vi "Check_Execution_Row.vi"(0 "Execution Row":T1 {"Row Duration (mins)" format="%#.1f"; "Row No" min=0; "Trace Gas Concentration (%)" min=0.0 format="%#.2f"; "Emission Rate (l/min)" format="%#.2f"; "Tunnel Speed" format="%#.2f"; "Start X" format="%#.2f"; "Start Y" format="%#.2f"; "Start Z" format="%#.2f"; "End X" format="%#.2f"; "End Y" format="%#.2f"; "End Z" format="%#.2f"; "Averaging time (min)" min=0.0 format="%#.2f"}, 3 "Synchronization Start No":i32=1 min=1 max=100, 4 "Row Index":i32, 5 "Max Tunnel Speed":dbl format="%.2f") -> (6 "Editted Row":bool, 7 "Execution Row Out":T1 {"Row Duration (mins)" format="%#.1f"; "Row No" min=0; "Trace Gas Concentration (%)" min=0.0 format="%#.2f"; "Emission Rate (l/min)" format="%#.2f"; "Tunnel Speed" format="%#.2f"; "Start X" format="%#.2f"; "Start Y" format="%#.2f"; "Start Z" format="%#.2f"; "End X" format="%#.2f"; "End Y" format="%#.2f"; "End Z" format="%#.2f"; "Averaging time (min)" min=0.0 format="%#.2f"}, 9 "Continue?":bool, 10 "Error Comments":string)   [LabVIEW 2011]
uses:
  Traverse_cluster.ctl
  Spacing.ctl
  Controls/Multi_run_mode.ctl
  Controls/User_Specific_mode.ctl
  Controls/Tunnel_Coordinates.ctl
  ADAM Client/Sub VIs/ADAM Controls/Channel_names.ctl
  Globals/Extra_Commands_Global.vi
  Globals/Constants_global.vi
  Globals/Trav_pos_global.vi
panel:
  out "Fixed Axis":bool[](array[boolean])
  out "Filenames":string[](array[string])
  out "Current Sync Number":i32
  out "Checks":string[](array[string])
  in  "Edit in Excel":bool
  in  "OK":bool
  # "X           Y            Z"
  # "Start"
  # "End"
  # "X           Y            Z"
  # "Start"
  # "End"
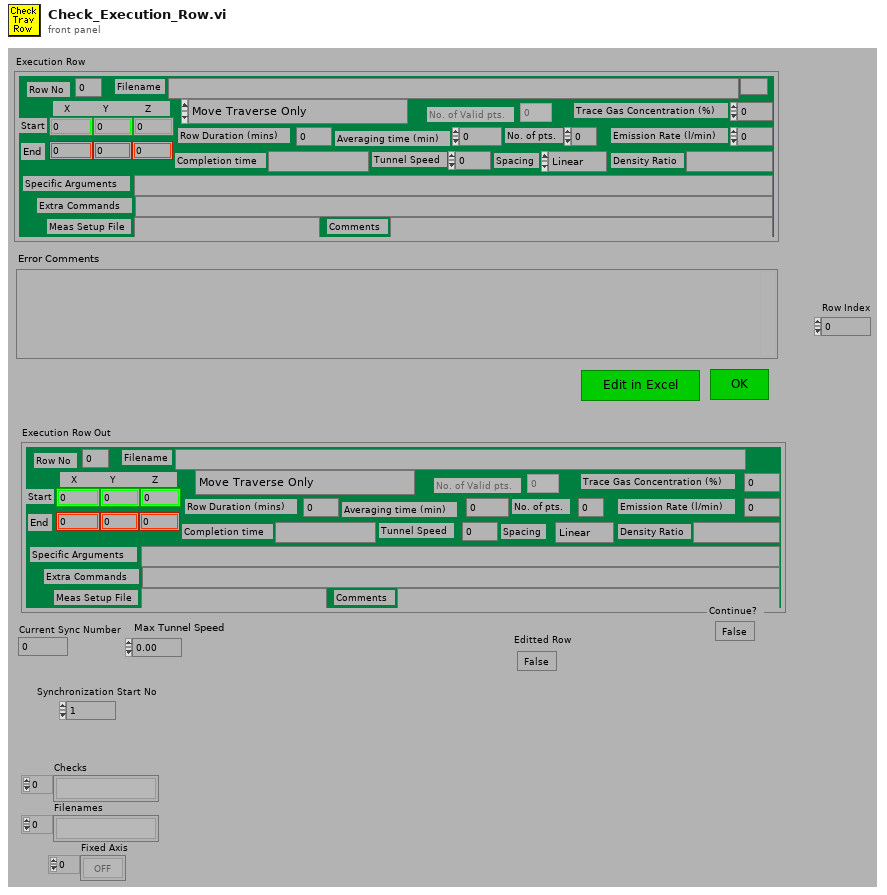
[diagram p1: front panel]
types:
  T1 = typedef "Traverse_cluster.ctl" = cluster{"Start X":dbl, "Start Y":dbl, "Start Z":dbl, "End X":dbl, "End Y":dbl, "End Z":dbl, "No. of pts.":i32, "Spacing":T2, "Filename":path, "Tunnel Speed":dbl, "Averaging time (min)":dbl, "Extra Commands":string, "Specific Arguments":string, "Emission Rate (l/min)":dbl, "Trace Gas Concentration (%)":dbl, "Density Ratio":string, "Comments":string, "Row No":i32, "Row Type Selector":T3, "Completion time":string, "Row Duration (mins)":dbl, "No. of Valid pts.":i32, "Meas Setup File":string}
  T2 = typedef "Spacing.ctl" = enum16{"Linear", "Log", "Gauss", "Specified", "N/A"}
  T3 = typedef "Multi_run_mode.ctl" = enum16{"Move Traverse Only", "Set Tunnel Speed Only", "Set Source Only", "Set Measurement Conditions", "Single Measurement", "Vertical Profile", "Lateral Profile", "Longitudinal Profile", "Explore Volume", "Multi-Axis Profile", "Auto Calibrate", "Meas Fast FID Bkgnd", "Check Beam Power", "Scanning Valve Measurement", "Run VI Named:", "Set ADAM Ch", "Wait (minutes)", "Send Message", "Synchronize With:", "Fall Back to this Row", "Turn Off Row Repeating", "Blank Row"}
  T4 = enum16{"All Channel Names", "Valid Channel Names"}
  T5 = typedef "User_Specific_mode.ctl" = enum16{"Check VI only", "Run VI"}
  T6 = typedef "Tunnel_Coordinates.ctl" = enum16{"Work in Tunnel Coordinates", "Work in Model Coordinates"}
  T7 = enum16{"Zero or one", "One", "Zero or more", "One or more"}
  T8 = typedef "Channel_names.ctl" = enum16{"Active Only", "Active + Off", "All Channels"}
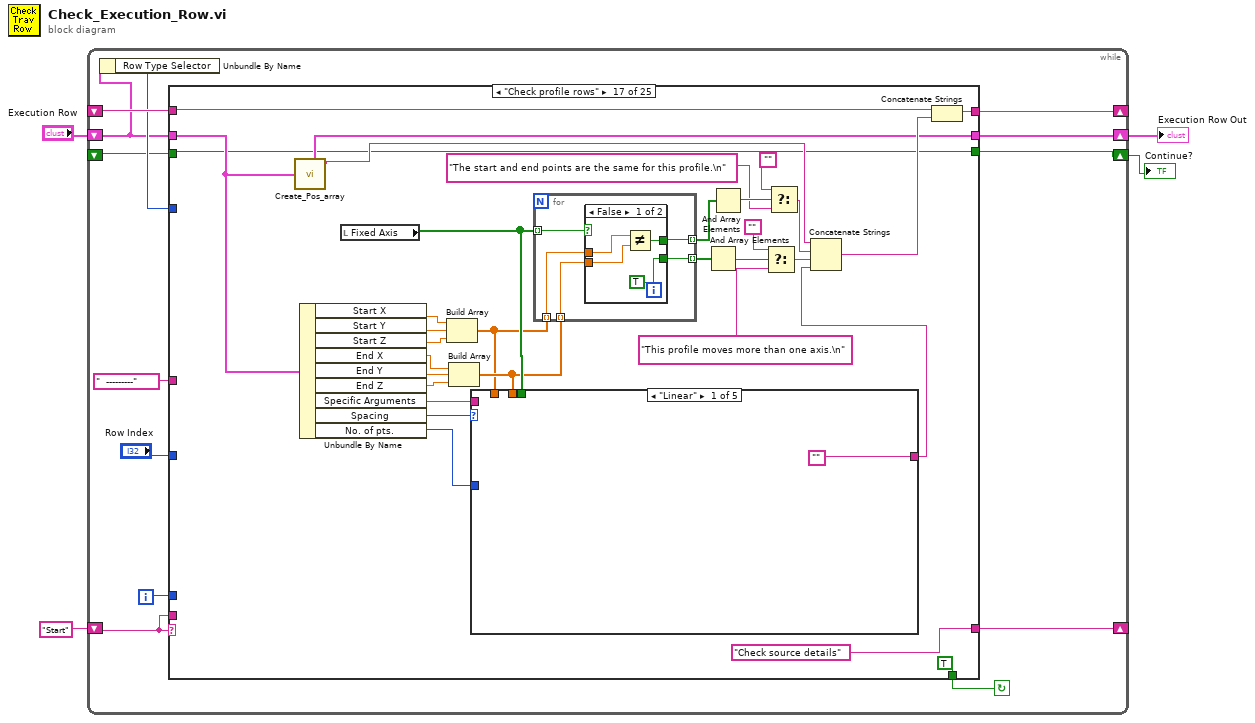
[diagram p0: block diagram]
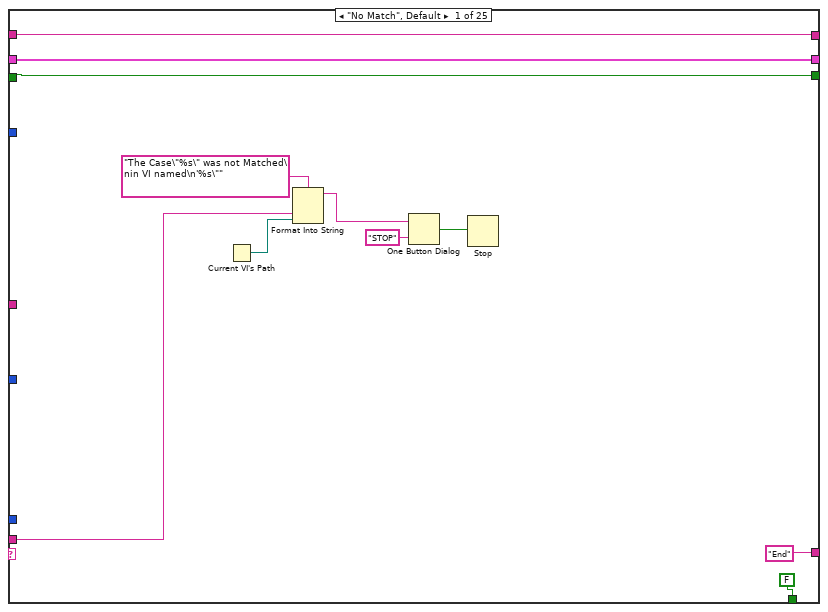
[diagram p2: hidden frame]
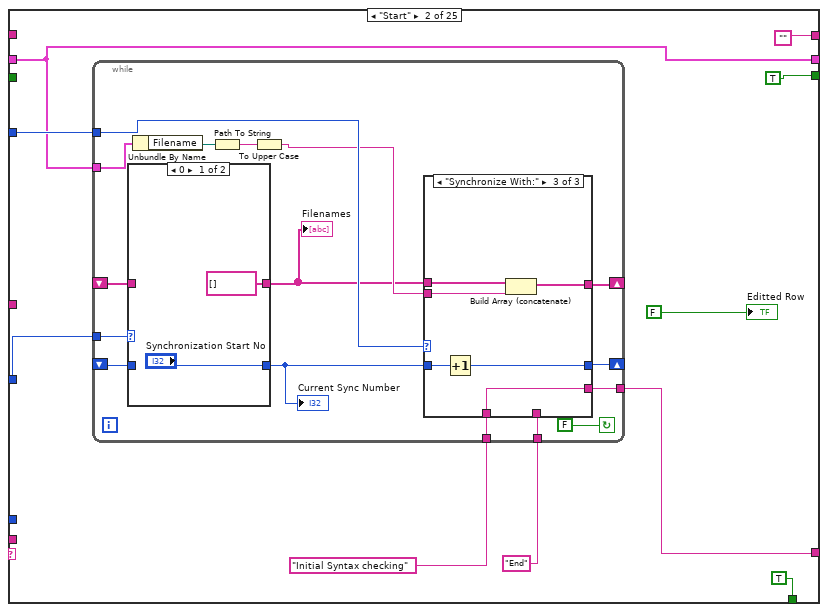
[diagram p3: hidden frame]
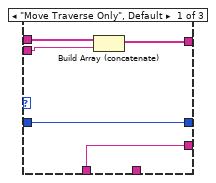
[diagram p5: hidden frame]
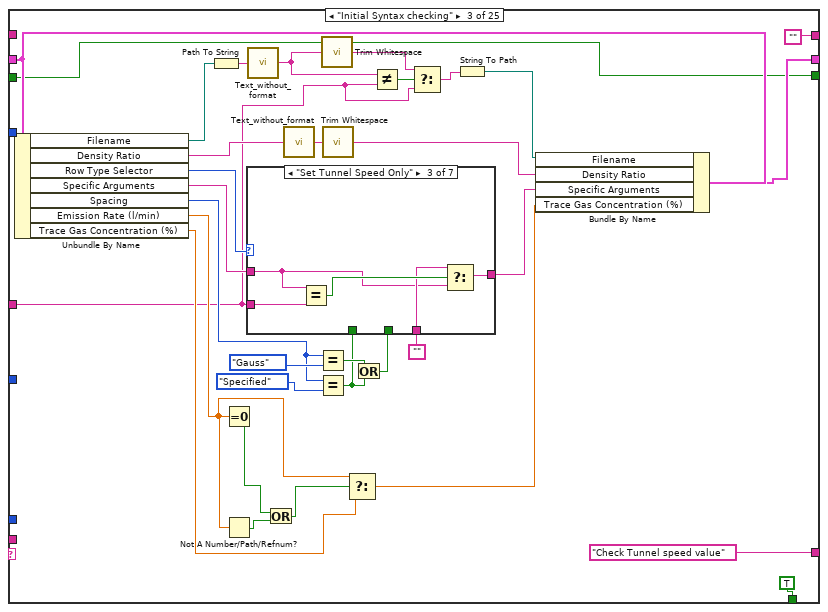
[diagram p7: hidden frame]
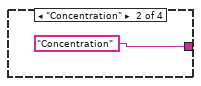
[diagram p10: hidden frame]
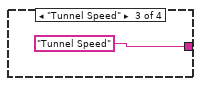
[diagram p11: hidden frame]
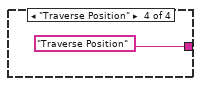
[diagram p12: hidden frame]
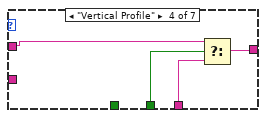
[diagram p13: hidden frame]
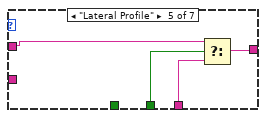
[diagram p14: hidden frame]
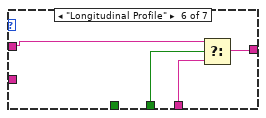
[diagram p15: hidden frame]
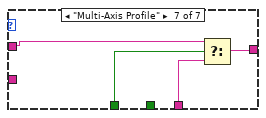
[diagram p16: hidden frame]
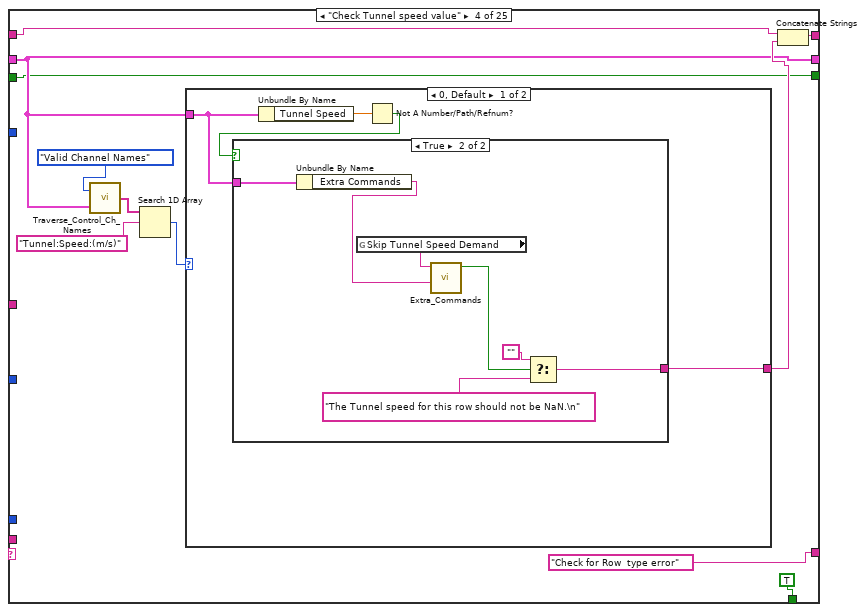
[diagram p17: hidden frame]
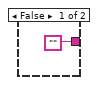
[diagram p18: hidden frame]
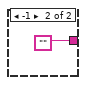
[diagram p19: hidden frame]
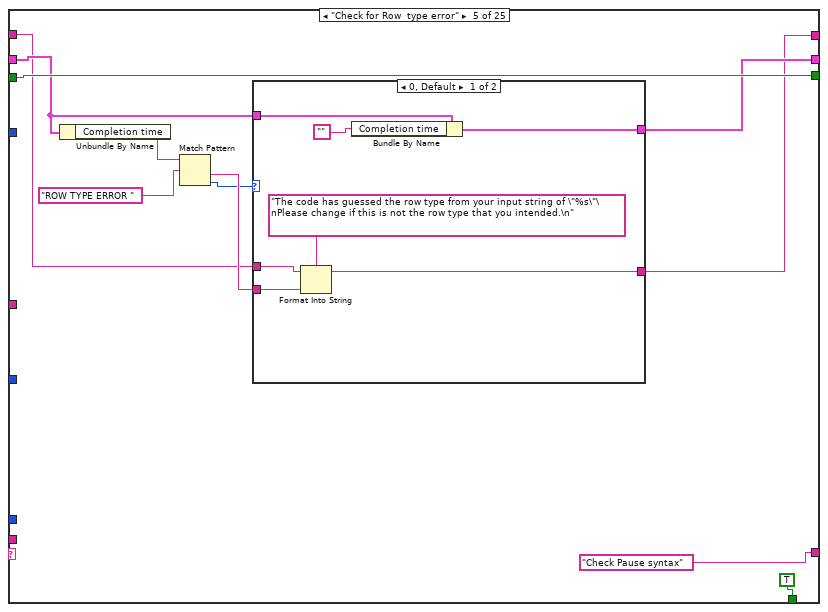
[diagram p20: hidden frame]
diagram:
  n1 = while {
    shift-left: _ -> [w16]
    shift-right: [w17] -> _
    shift-left: "Start" -> [w9]
    shift-right: [w14] -> _
    shift-right: [w8] -> w2
    shift-left: "Execution Row" -> [w5]
    shift-right: [w7] -> w1
    shift-left: _ -> [w6]
    i -> [w10]
    stop <- w15 continue-if-true
    n2 = Unbundle By Name(w5) -> ("Row Type Selector"=w12:T3)
    n3 = case shown="\"Check profile rows\"" w9 {
      tunnel: w5 -> [w22 w32 w100 w137 w161 w191 w205 w248 w278 w334 w366 w374 w413 w744 w844 w881 w903 w987 w1019 w1029 w1098 _ w1137 w1144 w1154]
      tunnel: "  ---------" ("f") -> [_ _ w74 _ _ w195 _ _ _ _ _ _ _ _ _ _ _ _ _ _ _ _ _ _ _]
      tunnel: "Row Index" -> [_ w36 _ _ _ _ w202 _ _ _ _ _ w407 _ _ _ _ _ _ _ _ _ w1138 _ w1153]
      tunnel: [w21 "" "" w138 w158 w183 w213 w253 w283 w336 w370 w379 w417 w749 w854 w887 w928 w985 w1023 w1030 w1104 w1115 w1139 w1149 w1156] -> w17
      tunnel: w12 -> [_ w35 _ _ _ _ _ _ _ _ _ w377 w416 w745 w842 _ _ _ _ w1034 _ _ _ _ _]
      tunnel: w16 -> [w21 _ _ w139 w159 w185 w214 w254 w284 w336 w369 w380 w418 w749 w855 w888 w929 w985 w1024 w1035 w1104 w1115 w1139 w1149 w1156]
      tunnel: [FALSE TRUE TRUE TRUE TRUE TRUE TRUE TRUE TRUE TRUE TRUE TRUE TRUE TRUE TRUE TRUE TRUE TRUE TRUE w1026 TRUE TRUE TRUE TRUE FALSE] -> w15
      tunnel: ["End" w33 "Check Tunnel speed value" ("f") "Check for Row  type error" ("f") "Check Pause syntax" ("f") w188 "Check Traverse Setup Name" ("f") "Check IF command" ("f") "Check Measurement Setup?" ("f") w338 "Check Maximum tunnel speed" ("f") "Row type specific check" ("f") w414 "Check for position NaNs" ("f") w845 "Check source details" ("t") "Check source details" ("f") w982 "check entered filename etc" ("f") w1032 "What to do next?" ("f") w1113 "Initial Syntax checking" "End" "End"] -> w14
      tunnel: w10 -> [_ _ _ _ _ _ _ _ _ _ _ _ _ _ _ _ _ _ _ _ _ _ _ _ _]
      tunnel: w9 -> [w23 _ _ _ _ _ _ _ _ _ _ _ _ _ _ _ _ _ _ _ _ _ _ _ _]
      tunnel: [w22 w32 w77 w137 w162 w178 w204 w248 w278 w334 w365 w374 w408 w743 w844 w881 w902 w986 w1019 w1028 w1098 w1106 w1140 w1144 w1152] -> w8
      tunnel: [w18 TRUE w75 w136 w168 w179 w206 w245 w275 w340 w367 w372 w410 w741 w843 w880 w900 w990 w1017 w1026 w1097 w1105 w1134 w1143 w1150] -> w7
      tunnel: w6 -> [w18 _ w75 w136 w168 w179 w206 w245 w275 w340 w367 w372 w410 w741 w843 w880 w900 w990 w1017 _ w1097 _ w1134 w1143 w1150]
      frame "No Match", Default {
        n4 = Current VI's Path() -> (path=w24:path)
        n5 = Format Into String(format string="The Case\"%s\" was not Matched\nin VI named\n'%s\"" ("Format String"), w23, w24) -> (resulting string=w27:string)  [unwired: 2 in, 1 out]
        n6 = One Button Dialog(message=w27, button name ("OK")="STOP") -> (true=w25:bool)
        n7 = Stop(stop? (T)=w25) -> ()
      }
      frame "Start" {
        n8 = while {
          tunnel: "End" -> [w40]
          tunnel: "Initial Syntax checking" -> [w41]
          tunnel: [w42] -> w33
          tunnel: w32 -> [w49]
          shift-left: _ -> [w48]
          shift-right: [w47] -> _
          tunnel: w35 -> [w53]
          shift-left: _ -> [w52]
          shift-right: [w51] -> _
          tunnel: w36 -> [w54]
          stop <- FALSE continue-if-true
          n9 = case shown="0" w54 {
            tunnel: ["Synchronization Start No" w58] -> w50
            tunnel: w52 -> [_ w58]
            tunnel: w48 -> [_ w57]
            tunnel: [string[] [] w57] -> w43
            frame 0 {
            }
            frame 1, Default {
            }
          }
          "Current Sync Number" <- w50
          "Filenames" <- w43
          n10 = Unbundle By Name(w49) -> ("Filename"=w46:path)
          n11 = Path To String(path=w46) -> (string=w45:string)
          n12 = To Upper Case(1:w45) -> (0:w44:string)
          n13 = case shown="\"Synchronize With:\"" w53 {
            tunnel: w50 -> [w63 w66 w72]
            tunnel: [w63 w66 w71] -> w51
            tunnel: w44 -> [w61 _ w70]
            tunnel: w43 -> [w62 w65 w69]
            tunnel: [w60 w65 w68] -> w47
            tunnel: [w59 w64 w67] -> w42
            tunnel: w41 -> [w59 _ w67]
            tunnel: w40 -> [_ w64 _]
            frame "Move Traverse Only", Default {
              n14 = Build Array (concatenate)(w62, w61) -> (w60:string[])
            }
            frame "Blank Row" {
            }
            frame "Synchronize With:" {
              n15 = Increment(x=w72) -> (x+1=w71:i32)
              n16 = Build Array (concatenate)(w69, w70) -> (w68:string[])
            }
          }
        }
        "Editted Row" <- FALSE ("Editted Row")
      }
      frame "Initial Syntax checking" {
        n17 = Unbundle By Name(w100) -> ("Filename"=w73:path, "Density Ratio"=w79:string, "Row Type Selector"=w97:T3, "Specific Arguments"=w95:string, "Spacing"=w87:T2, "Emission Rate (l/min)"=w83:dbl, "Trace Gas Concentration (%)"=w93:dbl)
        n18 = Path To String(path=w73) -> (string=w81:string)
        n19 = Equal To 0?(x=w83) -> (x = 0?=w85:bool)
        n20 = Not A Number/Path/Refnum?(number/path/refnum=w83) -> (NaN/Path/Refnum?=w84:bool)
        n21 = call "Text_without_format.vi"("Input string"=w81) -> ("Output string"=w104:string)
        n22 = Or(x=w85, y=w84) -> (x .or. y?=w82:bool)
        n23 = call "Text_without_format.vi"("Input string"=w79) -> ("Output string"=w99:string)
        n24 = Equal?(x=w87, y=Spacing."Gauss" ("Spacing")) -> (x = y?=w89:bool)
        n25 = Equal?(x=w87, y=Spacing."Specified" ("Spacing")) -> (x = y?=w86:bool)
        n26 = call <vilib>:"Trim Whitespace.vi"("string"=w104) -> ("trimmed string"=w103:string)  [unwired: 1 in]
        n27 = call <vilib>:"Trim Whitespace.vi"("string"=w99) -> ("trimmed string"=w78:string)  [unwired: 1 in]
        n28 = Select(t=w83, s=w82, f=w93) -> (s? t:f=w92:dbl)
        n29 = Or(x=w89, y=w86) -> (x .or. y?=w88:bool)
        n30 = case shown="\"Set Tunnel Speed Only\"" w97 {
          tunnel: [w106 w108 w113 w119 w123 w127 w131] -> w96
          tunnel: w95 -> [w106 w107 w114 w121 w125 w129 w133]
          tunnel: "" -> [_ _ w115 w120 w124 w128 w132]
          tunnel: w88 -> [_ _ _ w118 w122 w126 _]
          tunnel: w86 -> [_ _ _ _ _ _ w130]
          tunnel: w74 -> [_ _ w117 _ _ _ _]
          frame "Move Traverse Only", Default {
          }
          frame "Auto Calibrate" {
            n31 = case shown="\"No Match\", Default" w107 {
              tunnel: [w109 "Concentration" "Tunnel Speed" "Traverse Position"] -> w108
              tunnel: w107 -> [w109 _ _ _]
              frame "No Match", Default {
              }
              frame "Concentration" {
              }
              frame "Tunnel Speed" {
              }
              frame "Traverse Position" {
              }
            }
          }
          frame "Set Tunnel Speed Only" {
            n32 = Equal?(x=w114, y=w117) -> (x = y?=w116:bool)
            n33 = Select(t=w115, s=w116, f=w114) -> (s? t:f=w113:string)
          }
          frame "Vertical Profile" {
            n34 = Select(t=w121, s=w118, f=w120) -> (s? t:f=w119:string)
          }
          frame "Lateral Profile" {
            n35 = Select(t=w125, s=w122, f=w124) -> (s? t:f=w123:string)
          }
          frame "Longitudinal Profile" {
            n36 = Select(t=w129, s=w126, f=w128) -> (s? t:f=w127:string)
          }
          frame "Multi-Axis Profile" {
            n37 = Select(t=w133, s=w130, f=w132) -> (s? t:f=w131:string)
          }
        }
        n38 = Not Equal?(x=w104, y=w74) -> (x != y?=w105:bool)
        n39 = Select(t=w103, s=w105, f=w74) -> (s? t:f=w102:string)
        n40 = String To Path(string=w102) -> (path=w80:path)
        n41 = Bundle By Name(cluster=w100, "Filename"=w80, "Density Ratio"=w78, "Specific Arguments"=w96, "Trace Gas Concentration (%)"=w92) -> (w77:T1)
      }
      frame "Check Tunnel speed value" {
        n42 = call "Traverse_Control_Ch_Names.vi"("Traverse line"=w137, "Mode"=T4."Valid Channel Names") -> ("Channel names"=w143:string[])
        n43 = Search 1D Array(1D array=w143, element="Tunnel:Speed:(m/s)" ("Label for value")) -> (index of element=w141:i32)  [unwired: 1 out]
        n44 = case shown="0, Default" w141 {
          tunnel: w137 -> [w146 _]
          tunnel: [w145 ""] -> w140
          frame 0, Default {
            n45 = Unbundle By Name(w146) -> ("Tunnel Speed"=w148:dbl)
            n46 = Not A Number/Path/Refnum?(number/path/refnum=w148) -> (NaN/Path/Refnum?=w147:bool)
            n47 = case shown="True" w147 {
              tunnel: w146 -> [_ w156]
              tunnel: ["" w150] -> w145
              frame False {
              }
              frame True {
                n48 = Unbundle By Name(w156) -> ("Extra Commands"=w154:string)
                n49 = global read "Extra_Commands_Global.vi" "Skip Tunnel Speed Demand"() -> (w155:string)
                n50 = call "Extra_Commands.vi"("String to Search"=w154, "Command"=w155) -> ("Command Found"=w153:bool)  [unwired: 1 in, 4 out]
                n51 = Select(t="", s=w153, f="The Tunnel speed for this row should not be NaN.\n") -> (s? t:f=w150:string)
              }
            }
          }
          frame -1 {
          }
        }
        n52 = Concatenate Strings(w139, w140) -> (w138:string)
      }
      frame "Check for Row  type error" {
        n53 = Unbundle By Name(w161) -> ("Completion time"=w164:string)
        n54 = Match Pattern(string=w164, regular expression="ROW TYPE ERROR " ("format string")) -> (after substring=w163:string, offset past match=w160:i32)  [unwired: 3 out]
        n55 = case shown="0, Default" w160 {
          tunnel: w163 -> [w175 _]
          tunnel: [w173 w177] -> w162
          tunnel: w161 -> [w172 w177]
          tunnel: [w170 w176] -> w158
          tunnel: w159 -> [w169 w176]
          frame 0, Default {
            n56 = Format Into String(format string="The code has guessed the row type from your input string of \"%s\"\nPlease change if this is not the row type that you intended.\n", initial string=w169, w175) -> (resulting string=w170:string)  [unwired: 1 in, 1 out]
            n57 = Bundle By Name(cluster=w172, "Completion time"="") -> (w173:T1)
          }
          frame -1 {
          }
        }
      }
      frame "Check Pause syntax" {
        n58 = Unbundle By Name(w191) -> ("Extra Commands"=w196:string)
        n59 = Not Equal?(x=w196, y=w195) -> (x != y?=w197:bool)
        n60 = Select(t=w196, s=w197, f="") -> (s? t:f=w193:string)
        n61 = call <vilib>:"Trim Whitespace.vi"("string"=w193) -> ("trimmed string"=w187:string)  [unwired: 1 in]
        n62 = Equal?(x=w187, y="") -> (x = y?=w189:bool)
        n63 = call "Pause_for_server_ch_val.vi"("Extra command string"=w187, "Simulate/Run"=User_Specific_mode."Check VI only") -> ("Extra command string Out"=w186:string, "Error Comments"=w184:string)
        n64 = Bundle By Name(cluster=w191, "Extra Commands"=w186) -> (w178:T1)
        n65 = Concatenate Strings(w185, w184) -> (w183:string)
        n66 = Select(t="Check Measurement Setup?", s=w189, f="Check Extra Commands") -> (s? t:f=w188:string)
      }
      frame "Check Extra Commands" {
        n67 = Unbundle By Name(w205) -> ("Extra Commands"=w207:string)
        n68 = for {
          N: 4 -> [_]
          tunnel: w207 -> [w222]
          shift-right: [w218] -> w210
          shift-left: "" -> [w219]
          i -> [w224]
          n69 = case shown="0, Default" w224 {
            tunnel: [w227 w229 w231 w233] -> w221
            tunnel: ["The Extra Command \"%s\" should have a numeric argument.\n" ("Format String") "The Extra Command \"%s\" should have a numeric argument.\n" ("Format String") "The Extra Command \"%s\" should have a numeric argument.\n" ("Format String") "The Extra Command \"%s\" should have a numeric argument.\n" ("Format String")] -> w216
            frame 0, Default {
              n70 = global read "Extra_Commands_Global.vi" "Coil Analysis time (s)"() -> (w227:string)
            }
            frame 1 {
              n71 = global read "Extra_Commands_Global.vi" "Estimated Av Csample/Csource"() -> (w229:string)
            }
            frame 2 {
              n72 = global read "Extra_Commands_Global.vi" "Establish Exp Conditions (s)"() -> (w231:string)
            }
            frame 3 {
              n73 = global read "Extra_Commands_Global.vi" "Minutes Before Repeating Row"() -> (w233:string)
            }
          }
          n74 = call "Extra_Commands.vi"("String to Search"=w222, "Command"=w221) -> ("String Value"=w223:string, "Command Found"=w225:bool)  [unwired: 1 in, 3 out]
          n75 = case shown="False" w225 {
            tunnel: w223 -> [_ w242]
            tunnel: w221 -> [_ w240]
            tunnel: [w234 w237] -> w220
            tunnel: "" -> [w234 w236]
            tunnel: w216 -> [_ w235]
            frame False {
            }
            frame True {
              n76 = Decimal String To Number(string=w242) -> (offset past number=w241:i32)  [unwired: 3 out]
              n77 = Equal To 0?(x=w241) -> (x = 0?=w239:bool)
              n78 = Format Into String(format string=w235, w240) -> (resulting string=w238:string)  [unwired: 2 in, 1 out]
              n79 = Select(t=w238, s=w239, f=w236) -> (s? t:f=w237:string)
            }
          }
          n80 = Concatenate Strings(w220, w219) -> (w218:string)
        }
        n81 = call "Trav_Prog_Extra_Commands.vi"() -> ("Extra Commands Array"=w208:string[])  [unwired: 2 out]
        n82 = call "Valid_Extra_Command.vi"("Extra Commands string"=w207, "Valid Commands Array"=w208) -> ("Output String"=w212:string, "Extra Commands string Out"=w203:string)  [unwired: 3 out]
        n83 = Bundle By Name(cluster=w205, "Extra Commands"=w203) -> (w204:T1)
        n84 = call "Skip_If Sd_Error_Below.vi"("String to Search"=w203, "Simulate/Run"=User_Specific_mode."Check VI only", "Measurement setup Applied?"=FALSE, "Row Number"=w202) -> ("Error String"=w199:string)  [unwired: 1 in, 4 out]
        n85 = Concatenate Strings(w214, w212, w210, w199) -> (w213:string)
      }
      frame "Check Traverse Setup Name" {
        n86 = Unbundle By Name(w248) -> ("Extra Commands"=w244:string)
        n87 = global read "Extra_Commands_Global.vi" "!Traverse Setup"() -> (w251:string)
        n88 = call "Extra_Commands.vi"("String to Search"=w244, "Command"=w251) -> ("String Value"=w249:string, "Command Found"=w250:bool)  [unwired: 1 in, 3 out]
        n89 = case shown="True" w250 {
          tunnel: w249 -> [_ w261]
          tunnel: [w255 w258] -> w246
          tunnel: "" -> [w255 w257]
          frame False {
          }
          frame True {
            n90 = global read "Constants_global.vi" "Traverse folder"() -> (w256:path)
            n91 = List Folder(path=w256) -> (folder names=w259:string[])  [unwired: 1 in, 5 out]
            n92 = Search 1D Array(1D array=w259, element=w261) -> (index of element=w262:i32)  [unwired: 1 out]
            n93 = Greater Or Equal To 0?(x=w262) -> (x >= 0?=w260:bool)
            n94 = case shown="False" w260 {
              tunnel: w261 -> [w267 _]
              tunnel: w259 -> [w264 _]
              tunnel: [w263 w272] -> w258
              tunnel: w257 -> [_ w272]
              frame False {
                n95 = Format Into String(format string="%s is not a valid Travese setup. Valid option are:", w267) -> (resulting string=w265:string)  [unwired: 2 in, 1 out]
                n96 = for {
                  shift-right: [w269] -> w263
                  shift-left: w265 -> [w270]
                  tunnel: w264 -> [w271] mode=indexing
                  w268 = "  " ("Substring")
                  n97 = Concatenate Strings(w270, w268, w271, w268) -> (w269:string)
                }
              }
              frame True {
              }
            }
          }
        }
        n98 = Concatenate Strings(w254, w246) -> (w253:string)
      }
      frame "Check IF command" {
        n99 = Unbundle By Name(w278) -> ("Extra Commands"=w274:string)
        n100 = global read "Extra_Commands_Global.vi" "If Command"() -> (w281:string)
        n101 = call "Extra_Commands.vi"("String to Search"=w274, "Command"=w281) -> ("String Value"=w279:string, "Command Found"=w280:bool)  [unwired: 1 in, 3 out]
        n102 = case shown="True" w280 {
          tunnel: w279 -> [_ w290]
          tunnel: [w285 w289] -> w276
          tunnel: "" -> [w285 w287]
          frame False {
          }
          frame True {
            n103 = call "Get_array_values_fr_String.vi"("String Value"=w290) -> ("Numeric Array"=w286:dbl[], "String array"=w288:string[])
            n104 = Index Array(array=w288, index=0 ("Index")) -> (element=w291:string)
            n105 = case shown="\"Global Value Between\"" w291 {
              tunnel: w290 -> [w296 _ _ _]
              tunnel: [w295 w321 w322 "The !If  command has not been recognised.\nExtra command Example:\n!IF = Time Between;10:45;and;14:00;Execute Row (or) Skip Row\n\n!IF = ADAM Channel Between;Channel Name; 0.5;1.0\n\n!IF = Global Value Between; 0.5;1.0" ("Error Comments")] -> w289
              tunnel: w288 -> [_ w312 w330 _]
              tunnel: w287 -> [_ w305 w323 _]
              tunnel: w286 -> [_ _ _ _]
              frame "Time Between" {
                n106 = Get Date/Time In Seconds() -> (seconds since 1Jan1904=w293:timestamp)
                n107 = To Double Precision Float(number=w293) -> (double precision float=w294:dbl)
                n108 = call "If_Time_arguments.vi"("seconds since 1Jan1904"=w294, "String Value"=w296) -> ("Error Comments"=w295:string)  [unwired: 2 out]
              }
              frame "ADAM Channel Between" {
                n109 = Index Array(array=w312, index=1 ("Index")) -> (element=w315:string)
                n110 = Index Array(array=w312, index=2 ("Index")) -> (element=w311:string)
                n111 = Index Array(array=w312, index=3 ("Index")) -> (element=w310:string)
                n112 = Build Array(w315) -> (w317:string[])
                n113 = Decimal Digit?(1:w311) -> (0:w308:bool)
                n114 = Decimal Digit?(1:w310) -> (0:w309:bool)
                n115 = call "Get_Current_Scan_client.vi"("ADAM Ch Names"=w317) -> ("Numerical Values"=w319:dbl[])  [unwired: 3 out]
                n116 = And(x=w308, y=w309) -> (x .and. y?=w307:bool)
                n117 = Index Array(array=w319, index=0 ("Index")) -> (element=w320:dbl)
                n118 = Select(t=w305, s=w307, f="you must give two limits\n") -> (s? t:f=w301:string)
                n119 = Not A Number/Path/Refnum?(number/path/refnum=w320) -> (NaN/Path/Refnum?=w304:bool)
                n120 = Select(t="Invalid ADAM Channel Name\n", s=w304, f=w305) -> (s? t:f=w302:string)
                n121 = Concatenate Strings(w302, w301) -> (w299:string)
                n122 = Concatenate Strings(w299, "Extra command Example:\n!IF = ADAM Channel Between;Channel Name; 0.5;1.0") -> (w298:string)
                n123 = Empty String/Path?(string/path=w299) -> (empty?=w300:bool)
                n124 = Select(t=w305, s=w300, f=w298) -> (s? t:f=w321:string)
              }
              frame "Global Value Between" {
                n125 = Index Array(array=w330, index=1 ("Index")) -> (element=w329:string)
                n126 = Index Array(array=w330, index=2 ("Index")) -> (element=w328:string)
                n127 = Decimal Digit?(1:w329) -> (0:w326:bool)
                n128 = Decimal Digit?(1:w328) -> (0:w327:bool)
                n129 = And(x=w326, y=w327) -> (x .and. y?=w325:bool)
                n130 = Select(t=w323, s=w325, f="The Extra command IF statement must have two numerical values for the limits\n\nExtra command Example:\n!IF = Global Value Between; 0.5;1.0") -> (s? t:f=w322:string)
              }
              frame "No Match", Default {
              }
            }
          }
        }
        n131 = Concatenate Strings(w284, w276) -> (w283:string)
      }
      frame "Check Measurement Setup?" {
        n132 = Unbundle By Name(w334) -> ("Row Type Selector"=w339:T3, "Specific Arguments"=w337:string)
        n133 = case shown="\"Lateral Profile\"" w339 {
          tunnel: ["Check Measurement Setup" ("t") "Check Measurement Setup" ("t") "Check Measurement Setup" ("t") "Check Measurement Setup" ("t") "Check Measurement Setup" ("t") "Check Measurement Setup" ("t") "Check Measurement Setup" ("t") "Check Measurement Setup" ("t") "Check Measurement Setup" ("t") "Check Measurement Setup" ("t") w352 w361] -> w338
          tunnel: w337 -> [_ _ _ _ _ _ _ _ _ _ w359 _]
          tunnel: "Check Maximum tunnel speed" ("f") -> [_ _ _ _ _ _ _ _ _ _ w353 w361]
          tunnel: w334 -> [_ _ _ _ _ _ _ _ _ _ w356 _]
          frame "Lateral Profile" {
          }
          frame "Longitudinal Profile" {
          }
          frame "Explore Volume" {
          }
          frame "Multi-Axis Profile" {
          }
          frame "Vertical Profile" {
          }
          frame "Single Measurement" {
          }
          frame "Scanning Valve Measurement" {
          }
          frame "Auto Calibrate" {
          }
          frame "Meas Fast FID Bkgnd" {
          }
          frame "Check Beam Power" {
          }
          frame "Run VI Named:" {
            n134 = Match Pattern(string=w359, regular expression=";") -> (before substring=w358:string)  [unwired: 4 out]
            n135 = call <vilib>:"Trim Whitespace.vi"("string"=w358) -> ("trimmed string"=w357:string)  [unwired: 1 in]
            n136 = call "Run_VI_Named_specific.vi"("Run VI Named String"=w357, "Multi Run Row"=w356) -> ("Check Meas Setup?"=w355:bool)  [unwired: 9 out]
            n137 = Select(t="Check Measurement Setup", s=w355, f=w353) -> (s? t:f=w352:string)
          }
          frame "Set Tunnel Speed Only", Default {
          }
        }
      }
      frame "Check Measurement Setup" {
        n138 = Unbundle By Name(w366) -> ("Meas Setup File"=w364:string)
        n139 = call "Check_Measurement_Setups.vi"("Measurement Setup String"=w364) -> ("Measurement Setup String Out"=w363:string, "Error Comments"=w362:string)
        n140 = Bundle By Name(cluster=w366, "Meas Setup File"=w363) -> (w365:T1)
        n141 = Concatenate Strings(w369, w362) -> (w370:string)
      }
      frame "Check Maximum tunnel speed" {
        n142 = case shown="\"Set Tunnel Speed Only\", Default" w377 {
          tunnel: w374 -> [w399 _]
          tunnel: [w390 FALSE] -> w376
          tunnel: [w389 0.0] -> w375
          frame "Auto Calibrate" {
            n143 = Unbundle By Name(w399) -> ("Specific Arguments"=w398:string)
            n144 = call "Get_array_values_fr_String.vi"("String Value"=w398) -> ("Numeric Array"=w392:dbl[], "String array"=w397:string[])
            n145 = Index Array(array=w397, index=0 ("Index")) -> (element=w395:string)
            n146 = Equal?(x=w395, y="Tunnel Speed" ("Output Array")) -> (x = y?=w390:bool)
            n147 = Array Subset(array=w392, index=1 ("Array Index")) -> (w391:dbl[])  [unwired: 1 in]
            n148 = Array Max & Min(array=w391) -> (max value=w389:dbl)  [unwired: 3 out]
          }
          frame "Set Tunnel Speed Only", Default {
          }
        }
        n149 = case shown="False" w376 {
          tunnel: [w387 w388] -> w384
          tunnel: w374 -> [w386 _]
          tunnel: w375 -> [_ w388]
          frame False {
            n150 = Unbundle By Name(w386) -> ("Tunnel Speed"=w387:dbl)
          }
          frame True {
          }
        }
        n151 = Greater?(x=w384, y="Max Tunnel Speed") -> (0:w382:bool)
        n152 = Not A Number/Path/Refnum?(number/path/refnum=w384) -> (NaN/Path/Refnum?=w383:bool)
        n153 = Compound Arithmetic op=AND(invert w383, w382) -> (w381:bool)
        n154 = case shown="False" w381 {
          tunnel: w380 -> [w402 w404]
          tunnel: [w402 w403] -> w379
          tunnel: "Max Tunnel Speed" -> [_ w406]
          frame False {
          }
          frame True {
            n155 = Format Into String(format string="The maximum allowable tunnel speed is %.2f m/s.\n" ("Format String"), initial string=w404, w406) -> (resulting string=w403:string)  [unwired: 1 in, 1 out]
          }
        }
      }
      frame "Row type specific check" {
        n156 = case shown="\"Auto Calibrate\"" w416 {
          tunnel: w413 -> [w427 w436 w440 w444 w449 w454 w461 w468 w479 w487 w513 w567 w574 w595 w623 w672 w700 w705 w709 w721 w725 w731]
          tunnel: [string[] [] string[] [] string[] [] string[] [] w450 w457 w464 w471 w484 w492 w521 w569 string[] [] w612 string[] [] w667 string[] [] string[] [] string[] [] string[] [] string[] [] string[] []] -> w415
          tunnel: [w421 "" "" "" "" "" "" "" w480 w489 w535 w563 w573 w607 w615 w683 w702 "" w711 "" "" w733] -> w419
          tunnel: [w430 w437 w441 w445 w448 w455 w462 w469 w478 w488 w520 w557 w572 w606 w626 w668 "check entered filename etc" "check entered filename etc" "check entered filename etc" "check entered filename etc" "check entered filename etc" "check entered filename etc"] -> w414
          tunnel: "Check source details" -> [_ w437 w441 _ _ _ _ _ _ _ _ w557 w572 w606 w625 w669 _ _ _ _ _ _]
          tunnel: "Sort out start and end positions" -> [_ _ _ _ _ w455 w462 w469 _ w488 w518 _ _ _ _ _ _ _ _ _ _ _]
          tunnel: "Check for Start NaNs" -> [w430 _ _ w445 w448 _ _ _ w478 _ w519 _ _ _ _ _ _ _ _ _ _ _]
          tunnel: [w426 w436 w440 w444 w449 w454 w461 w468 w479 w487 w499 w567 w582 w595 w622 w672 w700 w705 w709 w721 w725 w729] -> w408
          tunnel: w407 -> [_ _ _ _ _ _ _ _ _ _ _ _ _ _ w628 _ _ _ _ _ _ _]
          frame "Move Traverse Only" {
            n157 = Unbundle By Name(w427) -> ("Specific Arguments"=w428:string)
            n158 = call <vilib>:"Trim Whitespace.vi"("string"=w428) -> ("trimmed string"=w422:string)  [unwired: 1 in]
            n159 = Equal?(x=w422, y="No Backlash") -> (x = y?=w425:bool)
            n160 = Empty String/Path?(string/path=w422) -> (empty?=w424:bool)
            n161 = Or(x=w424, y=w425) -> (x .or. y?=w423:bool)
            n162 = case shown="True" w423 {
              tunnel: w422 -> [w433 _]
              tunnel: [w432 ""] -> w421
              frame False {
                n163 = Format Into String(format string="\"%s\" is an Incorrect Specific Argument. It should either be left blank or say \"No Backlash\"\n", w433) -> (resulting string=w432:string)  [unwired: 2 in, 1 out]
              }
              frame True {
              }
            }
            n164 = Bundle By Name(cluster=w427, "Specific Arguments"=w422) -> (w426:T1)
          }
          frame "Set Tunnel Speed Only" {
          }
          frame "Set Source Only" {
          }
          frame "Set Measurement Conditions" {
          }
          frame "Single Measurement" {
            n165 = Build Array("Averaging:Time:(mins)" ("Label for value"), "Filename:HD:Users" ("Label for value")) -> (w450:string[])
          }
          frame "Vertical Profile" {
            n166 = Build Array("Number:Of:Points" ("Label for value"), "Averaging:Time:(mins)" ("Label for value"), "Filename:HD:Users" ("Label for value")) -> (w457:string[])
          }
          frame "Lateral Profile" {
            n167 = Build Array("Number:Of:Points" ("Label for value"), "Averaging:Time:(mins)" ("Label for value"), "Filename:HD:Users" ("Label for value")) -> (w464:string[])
          }
          frame "Longitudinal Profile" {
            n168 = Build Array("Number:Of:Points" ("Label for value"), "Averaging:Time:(mins)" ("Label for value"), "Filename:HD:Users" ("Label for value")) -> (w471:string[])
          }
          frame "Explore Volume" {
            n169 = Unbundle By Name(w479) -> ("Specific Arguments"=w477:string)
            n170 = Build Array("Averaging:Time:(mins)" ("Label for value"), "Filename:HD:Users" ("Label for value")) -> (w484:string[])
            n171 = Fract/Exp String To Number(string=w477) -> (number=w476:dbl)  [unwired: 4 out]
            n172 = Greater Than 0?(x=w476) -> (x > 0?=w475:bool)
            n173 = Format Into String(format string="\"%s\" is an Incorrect Specific Argument. Please enter the radius of the volume in mm.\n", w477) -> (resulting string=w481:string)  [unwired: 2 in, 1 out]
            n174 = Select(t="", s=w475, f=w481) -> (s? t:f=w480:string)
          }
          frame "Multi-Axis Profile" {
            n175 = Unbundle By Name(w487) -> ("Spacing"=w490:T2)
            n176 = case shown="\"N/A\"" w490 {
              tunnel: ["" "You are not allowed to specify gaussian spacing for a Multi-Axis profile.\n" "You are not allowed to specify Log spacing for a Multi-Axis profile.\n" "\"N/A\" is not a valid point spacing.\n"] -> w489
              frame "Linear", Default {
              }
              frame "Gauss" {
              }
              frame "Log" {
              }
              frame "N/A" {
              }
            }
            n177 = Build Array("Number:Of:Points" ("Label for value"), "Averaging:Time:(mins)" ("Label for value"), "Filename:HD:Users" ("Label for value")) -> (w492:string[])
          }
          frame "Auto Calibrate" {
            n178 = Unbundle By Name(w513) -> ("Filename"=w502:path, "Specific Arguments"=w534:string)
            n179 = call "Get_array_values_fr_String.vi"("String Value"=w534) -> ("Numeric Array"=w530:dbl[], "String array"=w517:string[])
            n180 = global read "Trav_pos_global.vi" "Work in Tunnel Coordinates?"() -> (w512:T6)
            n181 = Index Array(array=w517, index=0 ("Index")) -> (element=w516:string)
            n182 = Build Array("Tunnel Speed", "Traverse Position", "Concentration") -> (w515:string[])
            n183 = Build Array("Averaging:Time:(mins)" ("Label for value")) -> (w521:string[])
            n184 = Array Size(array=w530) -> (size(s)=w529:i32)
            n185 = call "Current_Filepath.vi"("Filename in"=w502, "Data Type"="Calibrations") -> ("Filename Out"=w500:path)  [unwired: 1 out]
            n186 = Equal?(x=w512, y=Tunnel_Coordinates."Work in Model Coordinates" ("Work in Tunnel Coordinates?")) -> (x = y?=w506:bool)
            n187 = Search 1D Array(1D array=w515, element=w516) -> (index of element=w507:i32)  [unwired: 1 out]
            n188 = Equal?(x=2, y=w507) -> (x = y?=w509:bool)
            n189 = case shown="1" w507 {
              tunnel: [w555 w556] -> w520
              tunnel: w519 -> [w555 _]
              tunnel: w518 -> [_ w556]
              frame 0, Default {
              }
              frame 1 {
              }
            }
            n190 = Less?(x=w529, y=3) -> (x < y?=w525:bool)
            n191 = Equal To 0?(x=w507) -> (x = 0?=w526:bool)
            n192 = And(x=w506, y=w509) -> (x .and. y?=w508:bool)
            n193 = Greater Or Equal To 0?(x=w507) -> (x >= 0?=w505:bool)
            n194 = Compound Arithmetic op=AND(w525, w526) -> (w524:bool)
            n195 = case shown="True" w508 {
              tunnel: w513 -> [w551 w553]
              tunnel: [w551 w552] -> w501
              frame False {
              }
              frame True {
                n196 = Bundle By Name(cluster=w553, "Comments"="WARNING POSITION IN TUNNEL COORDINATES!!") -> (w552:T1)
              }
            }
            n197 = Select(t="You need to enter the desired tunnel speeds in the \"Specfic Arguments\" Box   eg.  Tunnel Speed;1;2;3;4\n", s=w524, f="") -> (s? t:f=w522:string)
            n198 = call "Does_file_exist_(simple).vi"("Pathname"=w500) -> ("exists?"=w540:bool)
            n199 = case shown="False" w505 {
              tunnel: w515 -> [w542 _]
              tunnel: [w541 ""] -> w504
              frame False {
                n200 = for {
                  shift-right: [w547] -> w544
                  shift-left: "Incorrect Specific Argument. The options are: " -> [w548]
                  tunnel: w542 -> [w549] mode=indexing
                  w546 = "  " ("Substring")
                  n201 = Concatenate Strings(w548, w546, w549, w546) -> (w547:string)
                }
                n202 = Concatenate Strings(w544, "\r") -> (w541:string)
              }
              frame True {
              }
            }
            n203 = Select(t="", s=w540, f="The calibration file cannot be found.\n") -> (s? t:f=w536:string)
            n204 = Bundle By Name(cluster=w501, "Filename"=w500) -> (w499:T1)
            n205 = Concatenate Strings(w536, w522, w504) -> (w535:string)
          }
          frame "Meas Fast FID Bkgnd" {
            n206 = Unbundle By Name(w567) -> ("Specific Arguments"=w562:string)
            n207 = call "Get_array_values_fr_String.vi"("String Value"=w562) -> ("String array"=w561:string[])  [unwired: 1 out]
            n208 = Index Array(array=w561, index=0) -> (element=w559:string)
            n209 = Empty String/Path?(string/path=w559) -> (empty?=w565:bool)
            n210 = Build Array("Averaging:Time:(mins)" ("Label for value")) -> (w569:string[])
            n211 = Equal?(x=w559, y="Use Source Divertor Valve") -> (x = y?=w558:bool)
            n212 = Or(x=w565, y=w558) -> (x .or. y?=w564:bool)
            n213 = case shown="False" w564 {
              tunnel: ["Specific Argument should either be blank or\nUse Source Divertor Valve ; (wait time in seconds optional)" ""] -> w563
              frame False {
              }
              frame True {
              }
            }
          }
          frame "Check Beam Power" {
            n214 = Unbundle By Name(w574) -> ("Extra Commands"=w576:string, "Start X"=w581:dbl, "Start Y"=w579:dbl, "Start Z"=w580:dbl)
            n215 = global read "Extra_Commands_Global.vi" "Skip Traverse Position Demand"() -> (w577:string)
            n216 = call "Extra_Commands.vi"("String to Search"=w576, "Command"=w577) -> ("Command Found"=w575:bool)  [unwired: 1 in, 4 out]
            n217 = case shown="False" w575 {
              tunnel: w581 -> [w593 _]
              tunnel: w580 -> [w592 _]
              tunnel: w579 -> [w591 _]
              tunnel: "" -> [w588 w594]
              tunnel: [w587 w594] -> w573
              frame False {
                n218 = Build Array(w593, w591, w592) -> (w590:dbl[])
                n219 = Not A Number/Path/Refnum?(number/path/refnum=w590) -> (NaN/Path/Refnum?=w589:bool[])
                n220 = Or Array Elements(Boolean array=w589) -> (logical OR=w586:bool)
                n221 = Select(t="The start position is where the datum velocity measurement will be made. This should not contain NaNs.\n" ("f"), s=w586, f=w588) -> (s? t:f=w587:string)
              }
              frame True {
              }
            }
            n222 = Bundle By Name(cluster=w574, "Comments"="Start Position is the location of Datum Velocity Measurement") -> (w582:T1)
          }
          frame "Scanning Valve Measurement" {
            w608 = ext -0.5  # lo
            w609 = ext 47.5  # hi
            n223 = Unbundle By Name(w595) -> ("Specific Arguments"=w605:string)
            n224 = call "Get_array_values_fr_String.vi"("String Value"=w605) -> ("Numeric Array"=w604:dbl[], "String array"=w600:string[])
            n225 = Build Array("Averaging:Time:(mins)" ("Label for value"), "Filename:HD:Users" ("Label for value")) -> (w612:string[])
            n226 = Index Array(array=w600, index=0) -> (element=w599:string)
            n227 = Empty String/Path?(string/path=w599) -> (empty?=w597:bool)
            n228 = Index Array(array=w604, index=0) -> (element=w602:dbl)
            n229 = In Range and Coerce(upper limit=w609, x=w602, lower limit=w608) -> (In Range?=w598:bool)  [unwired: 1 out]
            n230 = Compound Arithmetic op=AND(invert w597, w598) -> (w596:bool)
            n231 = Select(t="", s=w596, f="Enter the scanning valve port number between 0 and 47 in the specific arguments box.\n") -> (s? t:f=w607:string)
          }
          frame "Set ADAM Ch" {
            n232 = Unbundle By Name(w623) -> ("Specific Arguments"=w634:string)
            n233 = while {
              shift-right: [w662] -> w630
              shift-left: _ -> [w655]
              shift-right: [w661] -> _
              shift-left: _ -> [w660]
              tunnel: w628 -> [w661]
              stop <- TRUE stop-if-true
              n234 = Array Size(array=w655) -> (size(s)=w659:i32)
              n235 = Less?(x=w661, y=w660) -> (x < y?=w657:bool)
              n236 = Equal To 0?(x=w659) -> (x = 0?=w658:bool)
              n237 = Or(x=w658, y=w657) -> (x .or. y?=w656:bool)
              n238 = case shown="True" w656 {
                tunnel: [w663 w664] -> w662
                tunnel: w655 -> [w663 _]
                frame False {
                }
                frame True {
                  n239 = call "Get_ADAM_Ch_names_client.vi"("Channel names set"=Channel_names."Active + Off") -> ("Ch names"=w664:string[])
                }
              }
            }
            n240 = call "Get_array_values_fr_String.vi"("String Value"=w634) -> ("String array"=w620:string[])  [unwired: 1 out]
            n241 = Index Array(array=w620, index=0) -> (element=w629:string)
            n242 = Search 1D Array(1D array=w630, element=w629) -> (index of element=w632:i32)  [unwired: 1 out]
            n243 = Index Array(array=w620, index=1) -> (element=w619:string)
            n244 = Empty String/Path?(string/path=w619) -> (empty?=w617:bool)
            n245 = Greater Or Equal To 0?(x=w632) -> (x >= 0?=w631:bool)
            n246 = Select(t="You have not specified a Value to Set the ADAM channel to.\nExample Specifice Argument:  ADAM_Ch_NAME  ;  10", s=w617, f="") -> (s? t:f=w615:string)
            n247 = case shown="False" w631 {
              tunnel: w630 -> [w651 _]
              tunnel: w629 -> [w649 _]
              tunnel: w628 -> [w647 _]
              tunnel: [w645 FALSE ("Cancel")] -> w627
              tunnel: w623 -> [w639 w652]
              tunnel: [w638 w652] -> w622
              tunnel: w619 -> [w636 _]
              frame False {
                n248 = Build Array(w649) -> (w648:string[])
                n249 = Format Into String(format string="Please Select the ADAM Channel that you want to set in row %d", w647) -> (resulting string=w646:string)  [unwired: 2 in, 1 out]
                n250 = call "Select_Strings.vi"("Available Ch names"=w651, "Message"=w646, "Selector mode"=T7."One", "Desired Ch names (in)"=w648) -> ("Cancel"=w645:bool, "Selected Channel Names"=w643:string[])  [unwired: 3 out]
                n251 = Index Array(array=w643, index=0) -> (element=w641:string)
                n252 = Concatenate Strings(w641, "  ;  " ("string"), w636) -> (w637:string)
                n253 = Bundle By Name(cluster=w639, "Specific Arguments"=w637) -> (w638:T1)
              }
              frame True {
              }
            }
            n254 = Select(t="Close Front Panel", s=w627, f=w625) -> (s? t:f=w626:string)
          }
          frame "Run VI Named:" {
            w677 = "Run_VI_Named_specific.vi"
            n255 = Unbundle By Name(w672) -> ("Specific Arguments"=w680:string)
            n256 = global read "Constants_global.vi" "Run VI Folder"() -> (w678:path)
            n257 = Match Pattern(string=w680, regular expression=";") -> (before substring=w681:string)  [unwired: 4 out]
            n258 = call <vilib>:"Trim Whitespace.vi"("string"=w681) -> ("trimmed string"=w673:string)  [unwired: 1 in]
            n259 = call "Run_VI_Named_specific.vi"("Run VI Named String"=w673, "Multi Run Row"=w672) -> ("Checks"=w667:string[], "Error String"=w666:string, "Check for start NaNs?"=w671:bool)  [unwired: 7 out]
            n260 = Select(t="Check for Start NaNs" ("Label for value"), s=w671, f=w669) -> (s? t:f=w668:string)
            n261 = Build Path(base path=w678, name or relative path=w673) -> (appended path=w684:path)
            n262 = Not Equal?(x=w673, y=w677) -> (x != y?=w676:bool)
            n263 = call "Does_file_exist_(simple).vi"("Pathname"=w684) -> ("exists?"=w675:bool)
            n264 = And(x=w675, y=w676) -> (x .and. y?=w674:bool)
            n265 = case shown="False" w674 {
              tunnel: [w691 ""] -> w679
              tunnel: w678 -> [w687 _]
              tunnel: w677 -> [w685 _]
              frame False {
                w689 = "\r"
                n266 = Build Array(w685) -> (w686:string[])
                n267 = call "List_files_in_order_of_age.vi"("Files to Hide"=w686, "Folder"=w687) -> ("file names"=w688:string[])
                n268 = for {
                  shift-right: [w695] -> w692
                  shift-left: "Cannot find the VI to run. Specific Argument options are:" -> [w696]
                  tunnel: w688 -> [w697] mode=indexing
                  w694 = "  " ("Substring")
                  n269 = Concatenate Strings(w696, w694, w697, w694) -> (w695:string)
                }
                n270 = Concatenate Strings(w692, w689, "Please place one of these strings in the \"Specific Argument\" field.", w689) -> (w691:string)
              }
              frame True {
              }
            }
            n271 = Concatenate Strings(w666, w679) -> (w683:string)
          }
          frame "Wait (minutes)" {
            n272 = Unbundle By Name(w700) -> ("Specific Arguments"=w701:string)
            n273 = call "Wait_Case_Arg.vi"("Specific Argument"=w701) -> ("Error Comments"=w702:string)  [unwired: 1 in, 4 out]
          }
          frame "Send Message" {
          }
          frame "Synchronize With:" {
            n274 = local read "Current Sync Number"() -> (w710:i32)
            n275 = call "Synchronize_Prog_Arg.vi"("Execution Row"=w709) -> ("Error Comments"=w712:string, "Sync No"=w718:i32)  [unwired: 3 out]
            n276 = Equal?(x=w718, y=w710) -> (x = y?=w717:bool)
            n277 = Format Into String(format string="This should be Synchroisation number %d.\n" ("Format String"), w710) -> (resulting string=w715:string)  [unwired: 2 in, 1 out]
            n278 = Select(t="", s=w717, f=w715) -> (s? t:f=w713:string)
            n279 = Concatenate Strings(w713, w712) -> (w711:string)
          }
          frame "Fall Back to this Row" {
          }
          frame "Turn Off Row Repeating" {
          }
          frame "Blank Row" {
            n280 = Unbundle By Name(w731) -> ("Comments"=w737:string)
            n281 = Match Pattern(string=w737, regular expression="(No Match Info)") -> (before substring=w730:string, after substring=w734:string)  [unwired: 3 out]
            n282 = Empty String/Path?(string/path=w734) -> (empty?=w735:bool)
            n283 = Bundle By Name(cluster=w731, "Comments"=w730) -> (w729:T1)
            n284 = Select(t=w734, s=w735, f="The Row Type Selector \"%s\" was not matched. Please select the desired type.\n") -> (s? t:f=w733:string)
          }
        }
        "Checks" <- w415
        n285 = Concatenate Strings(w418, w419) -> (w417:string)
      }
      frame "Sort out start and end positions" {
        n286 = Unbundle By Name(w744) -> ("Start X"=w756:dbl, "Start Y"=w755:dbl, "Start Z"=w754:dbl, "End X"=w753:dbl, "End Y"=w752:dbl, "End Z"=w751:dbl, "Extra Commands"=w740:string)
        n287 = call "Which_Trav_Setup.vi"("Extra Command String"=w740) -> ("Traverse Setup"=w739:string)
        n288 = call "Rig_Pict_Display_Pref.vi"("Traverse Name"=w739) -> ("Which Axis is vertical?"=w750:enum16{"X Axis", "Y Axis", "Z Axis"})  [unwired: 7 out]
        n289 = case shown="\"Auto Calibrate\"" w745 {
          tunnel: [w796 FALSE w812 w825 FALSE] -> w759
          tunnel: [w795 FALSE w811 w824 FALSE] -> w758
          tunnel: [w794 FALSE w810 w823 FALSE] -> w757
          tunnel: w750 -> [w793 _ w809 w822 _]
          frame "Vertical Profile" {
            n290 = case shown="\"X Axis\"" w793 {
              tunnel: [FALSE TRUE TRUE] -> w796
              tunnel: [TRUE FALSE TRUE] -> w795
              tunnel: [TRUE TRUE FALSE] -> w794
              frame "X Axis" {
              }
              frame "Y Axis" {
              }
              frame "Z Axis" {
              }
            }
          }
          frame "Auto Calibrate" {
          }
          frame "Lateral Profile" {
            n291 = case shown="\"Y Axis\"" w809 {
              tunnel: [TRUE TRUE TRUE] -> w812
              tunnel: [TRUE TRUE FALSE] -> w811
              tunnel: [FALSE FALSE TRUE] -> w810
              frame "X Axis" {
              }
              frame "Y Axis" {
              }
              frame "Z Axis" {
              }
            }
          }
          frame "Longitudinal Profile" {
            n292 = case shown="\"Y Axis\"" w822 {
              tunnel: [FALSE FALSE FALSE] -> w825
              tunnel: [TRUE TRUE TRUE] -> w824
              tunnel: [TRUE TRUE TRUE] -> w823
              frame "X Axis" {
              }
              frame "Y Axis" {
              }
              frame "Z Axis" {
              }
            }
          }
          frame "Multi-Axis Profile", Default {
          }
        }
        n293 = Build Array(w756, w755, w754) -> (w747:dbl[])
        n294 = Build Array(w753, w752, w751) -> (w746:dbl[])
        n295 = Build Array(w759, w758, w757) -> (w748:bool[])
        "Fixed Axis" <- w748
        n296 = for {
          tunnel: w748 -> [w766] mode=indexing
          tunnel: w747 -> [w765] mode=indexing
          tunnel: w746 -> [w764] mode=indexing
          shift-right: [w761] -> w743
          shift-left: w744 -> [w762]
          i -> [w763]
          n297 = case shown="True" w766 {
            tunnel: w765 -> [_ w772]
            tunnel: w764 -> [_ w771]
            tunnel: w763 -> [_ w770]
            tunnel: w762 -> [w767 w769]
            tunnel: [w767 w768] -> w761
            frame False {
            }
            frame True {
              n298 = Not A Number/Path/Refnum?(number/path/refnum=w772) -> (NaN/Path/Refnum?=w773:bool)
              n299 = Not A Number/Path/Refnum?(number/path/refnum=w771) -> (NaN/Path/Refnum?=w775:bool)
              n300 = Exclusive Or(1:w775, 2:w773) -> (0:w774:bool)
              n301 = case shown="True" w774 {
                tunnel: w773 -> [_ w783]
                tunnel: w772 -> [_ w782]
                tunnel: w771 -> [_ w781]
                tunnel: w770 -> [_ w780]
                tunnel: w769 -> [w776 w779]
                tunnel: [w776 w778] -> w768
                frame False {
                }
                frame True {
                  n302 = Select(t=w781, s=w783, f=w782) -> (s? t:f=w777:dbl)
                  n303 = case shown="2" w780 {
                    tunnel: w779 -> [w786 w789 w792]
                    tunnel: [w785 w788 w791] -> w778
                    tunnel: w777 -> [w784 w787 w790]
                    frame 0, Default {
                      n304 = Bundle By Name(cluster=w786, "Start X"=w784, "End X"=w784) -> (w785:T1)
                    }
                    frame 1 {
                      n305 = Bundle By Name(cluster=w789, "Start Y"=w787, "End Y"=w787) -> (w788:T1)
                    }
                    frame 2 {
                      n306 = Bundle By Name(cluster=w792, "Start Z"=w790, "End Z"=w790) -> (w791:T1)
                    }
                  }
                }
              }
            }
          }
        }
      }
      frame "Check for position NaNs" {
        n307 = global read "Extra_Commands_Global.vi" "Skip Traverse Position Demand"() -> (w841:string)
        n308 = Unbundle By Name(w844) -> ("Extra Commands"=w840:string, "Start X"=w853:dbl, "Start Y"=w851:dbl, "Start Z"=w852:dbl, "End X"=w850:dbl, "End Y"=w849:dbl, "End Z"=w848:dbl)
        n309 = call "Extra_Commands.vi"("String to Search"=w840, "Command"=w841) -> ("Command Found"=w838:bool)  [unwired: 1 in, 4 out]
        n310 = case shown="False" w838 {
          tunnel: w853 -> [w868 _]
          tunnel: w852 -> [w867 _]
          tunnel: w851 -> [w866 _]
          tunnel: w850 -> [w865 _]
          tunnel: w849 -> [w864 _]
          tunnel: w848 -> [w863 _]
          tunnel: [w859 w869] -> w847
          tunnel: [w858 TRUE] -> w846
          tunnel: "" -> [w857 w869]
          frame False {
            n311 = Build Array(w868, w866, w867, w865, w864, w863) -> (w862:dbl[])
            n312 = Not A Number/Path/Refnum?(number/path/refnum=w862) -> (NaN/Path/Refnum?=w861:bool[])
            n313 = Or Array Elements(Boolean array=w861) -> (logical OR=w858:bool)
            n314 = Select(t="Some of the Start and End positions are NaN.\n" ("f"), s=w858, f=w857) -> (s? t:f=w859:string)
          }
          frame True {
          }
        }
        n315 = case shown="\"Set Tunnel Speed Only\", Default" w842 {
          tunnel: w846 -> [_ w875]
          tunnel: ["Check source details" ("t") w874] -> w845
          frame "Multi-Axis Profile" {
          }
          frame "Set Tunnel Speed Only", Default {
            n316 = Select(t="Check source details", s=w875, f="Check profile rows") -> (s? t:f=w874:string)
          }
        }
        n317 = Concatenate Strings(w855, w847) -> (w854:string)
      }
      frame "Check for Start NaNs" {
        n318 = Unbundle By Name(w881) -> ("Extra Commands"=w877:string, "Start X"=w886:dbl, "Start Y"=w884:dbl, "Start Z"=w885:dbl)
        n319 = global read "Extra_Commands_Global.vi" "Skip Traverse Position Demand"() -> (w878:string)
        n320 = call "Extra_Commands.vi"("String to Search"=w877, "Command"=w878) -> ("Command Found"=w876:bool)  [unwired: 1 in, 4 out]
        n321 = case shown="False" w876 {
          tunnel: w886 -> [w898 _]
          tunnel: w885 -> [w897 _]
          tunnel: w884 -> [w896 _]
          tunnel: "" -> [w893 w899]
          tunnel: [w891 w899] -> w882
          frame False {
            n322 = Build Array(w898, w896, w897) -> (w895:dbl[])
            n323 = Not A Number/Path/Refnum?(number/path/refnum=w895) -> (NaN/Path/Refnum?=w894:bool[])
            n324 = Or Array Elements(Boolean array=w894) -> (logical OR=w890:bool)
            n325 = Select(t="Some of the Start coordinates are NaN.\n" ("f"), s=w890, f=w893) -> (s? t:f=w891:string)
          }
          frame True {
          }
        }
        n326 = Concatenate Strings(w888, w882) -> (w887:string)
      }
      frame "Check profile rows" {
        n327 = call "Create_Pos_array.vi"("Traverse line"=w903) -> ("Traverse line Out"=w902:T1, "Error Messages"=w901:string)  [unwired: 7 out]
        n328 = Unbundle By Name(w903) -> ("Start X"=w927:dbl, "Start Y"=w926:dbl, "Start Z"=w925:dbl, "End X"=w924:dbl, "End Y"=w923:dbl, "End Z"=w922:dbl, "Specific Arguments"=w916:string, "Spacing"=w909:T2, "No. of pts."=w908:i32)
        n329 = local read "Fixed Axis"() -> (w907:bool[])
        n330 = Build Array(w927, w926, w925) -> (w905:dbl[])
        n331 = Build Array(w924, w923, w922) -> (w906:dbl[])
        n332 = case shown="\"Linear\"" w909 {
          tunnel: w916 -> [_ _ _ _ w962]
          tunnel: ["" w935 "\"N/A\" is not a valid point spacing.\n" "" w957] -> w915
          tunnel: w908 -> [_ _ _ _ w961]
          tunnel: w907 -> [_ w933 _ _ _]
          tunnel: w906 -> [_ w940 _ _ _]
          tunnel: w905 -> [_ w939 _ _ _]
          frame "Linear" {
          }
          frame "Log" {
            n333 = for {
              tunnel: w940 -> [w944] mode=indexing
              tunnel: w939 -> [w943] mode=indexing
              tunnel: [w942] -> w938 mode=indexing
              tunnel: w933 -> [w941] mode=indexing
              n334 = case shown="False" w941 {
                tunnel: w944 -> [w950 _]
                tunnel: w943 -> [w949 _]
                tunnel: [w945 FALSE] -> w942
                frame False {
                  w948 = 0.001 ("y")
                  n335 = Less?(x=w950, y=w948) -> (x < y?=w946:bool)
                  n336 = Less?(x=w949, y=w948) -> (x < y?=w947:bool)
                  n337 = Or(x=w946, y=w947) -> (x .or. y?=w945:bool)
                }
                frame True {
                }
              }
            }
            n338 = Or Array Elements(Boolean array=w938) -> (logical OR=w937:bool)
            n339 = Select(t="For log spacing, Start & End positions must be greater than 0.0001.", s=w937, f="") -> (s? t:f=w935:string)
          }
          frame "N/A" {
          }
          frame "Gauss" {
          }
          frame "Specified" {
            n340 = call "Get_array_values_fr_String.vi"("String Value"=w962) -> ("Numeric Array"=w956:dbl[])  [unwired: 1 out]
            n341 = Array Size(array=w956) -> (size(s)=w955:i32)
            n342 = Decrement(x=w955) -> (x-1=w954:i32)
            n343 = Equal?(x=w954, y=w961) -> (x = y?=w960:bool)
            n344 = Select(t="", s=w960, f="The No of points and No of Arguments do not match.\n") -> (s? t:f=w957:string)
          }
        }
        n345 = for {
          tunnel: w907 -> [w967] mode=indexing
          tunnel: w905 -> [w966] mode=indexing
          tunnel: w906 -> [w965] mode=indexing
          tunnel: [w964] -> w921 mode=indexing
          tunnel: [w963] -> w912 mode=indexing
          n346 = case shown="False" w967 {
            tunnel: w966 -> [w969 w975]
            tunnel: w965 -> [w970 w974]
            tunnel: [TRUE w973] -> w964
            tunnel: [w968 TRUE] -> w963
            frame False {
              n347 = Not Equal?(x=w969, y=w970) -> (x != y?=w968:bool)
            }
            frame True {
              n348 = Equal?(x=w975, y=w974) -> (x = y?=w973:bool)
            }
          }
        }
        n349 = And Array Elements(Boolean array=w921) -> (logical AND=w920:bool)
        n350 = And Array Elements(Boolean array=w912) -> (logical AND=w913:bool)
        n351 = Select(t="", s=w920, f="This profile moves more than one axis.\n") -> (s? t:f=w917:string)
        n352 = Select(t="", s=w913, f="The start and end points are the same for this profile.\n") -> (s? t:f=w911:string)
        n353 = Concatenate Strings(w901, w911, w917, w915) -> (w930:string)
        n354 = Concatenate Strings(w929, w930) -> (w928:string)
      }
      frame "Check source details" {
        n355 = Unbundle By Name(w987) -> ("Emission Rate (l/min)"=w989:dbl, "Density Ratio"=w979:string)  [unwired: 1 out]
        n356 = Empty String/Path?(string/path=w979) -> (empty?=w980:bool)
        n357 = Equal?(x=w979, y="---------" ("f")) -> (x = y?=w978:bool)
        n358 = Or(x=w980, y=w978) -> (x .or. y?=w977:bool)
        n359 = Greater Than 0?(x=w989) -> (x > 0?=w984:bool)
        n360 = And(x=w984, y=w977) -> (x .and. y?=w988:bool)
        n361 = case shown="True" w988 {
          tunnel: w987 -> [w992 w995]
          tunnel: [w992 w993] -> w986
          frame False {
          }
          frame True {
            (unwired) "The Density Ratio Box should contain either:\nCarrier 1 Only\nCarrier 2 Only\nor the relative density ratio of the mixed gas with respect to air" ("f")
            n362 = Bundle By Name(cluster=w995, "Density Ratio"="Carrier 1 Only") -> (w993:T1)
          }
        }
        n363 = Select(t="Check source detail 2", s=w984, f="check entered filename etc") -> (s? t:f=w982:string)
      }
      frame "Check source detail 2" {
        n364 = Unbundle By Name(w1019) -> ("Trace Gas Concentration (%)"=w1020:dbl, "Density Ratio"=w1021:string)
        n365 = To Upper Case(1:w1021) -> (0:w1004:string)
        n366 = To Upper Case(1:"Carrier 1 Only") -> (0:w1006:string)
        n367 = To Upper Case(1:"Carrier 2 Only") -> (0:w1005:string)
        n368 = In Range and Coerce(upper limit=ext 3.01 ("hi"), x=w1020, lower limit=ext 0.0 ("lo")) -> (In Range?=w1001:bool)  [unwired: 1 out]
        n369 = Equal?(x=w1004, y=w1006) -> (x = y?=w1011:bool)
        n370 = Equal?(x=w1004, y=w1005) -> (x = y?=w1010:bool)
        n371 = Fract/Exp String To Number(string=w1004) -> (number=w1012:dbl)  [unwired: 4 out]
        n372 = In Range and Coerce(upper limit=ext 10.0 ("hi"), x=w1012, lower limit=ext 0.05 ("lo")) -> (In Range?=w1009:bool)  [unwired: 1 out]
        n373 = Compound Arithmetic op=OR(w1011, w1010, w1009) -> (w996:bool)
        n374 = Select(t="", s=w1001, f="The Trace Gas Concentration must be within the range of 0 to 3%.\n") -> (s? t:f=w997:string)
        n375 = Select(t="", s=w996, f="The Density Ratio Box should contain either:\nCarrier 1 Only\nCarrier 2 Only\nor the relative density ratio of the mixed gas with respect to air") -> (s? t:f=w998:string)
        n376 = Concatenate Strings(w997, w998) -> (w1022:string)
        n377 = Concatenate Strings(w1024, w1022) -> (w1023:string)
      }
      frame "check entered filename etc" {
        n378 = local read "Checks"() -> (w1037:string[])
        n379 = for {
          tunnel: w1037 -> [w1044] mode=indexing
          tunnel: [w1049] -> w1038 mode=indexing
          tunnel: w1034 -> [w1048]
          shift-right: [w1046] -> w1028
          shift-left: w1029 -> [w1047]
          tunnel: [w1045] -> w1027 mode=indexing
          n380 = case shown="\"Filename:HD:Users\"" w1044 {
            tunnel: w1047 -> [w1051 w1059 w1081 w1096]
            tunnel: [w1052 w1062 w1087 w1092] -> w1049
            tunnel: w1048 -> [_ _ w1090 _]
            tunnel: [w1051 w1059 w1079 w1096] -> w1046
            tunnel: [TRUE ("cancelled") TRUE ("cancelled") w1074 TRUE ("cancelled")] -> w1045
            tunnel: w1044 -> [_ _ _ w1094]
            frame "Number:Of:Points" {
              n381 = Unbundle By Name(w1051) -> ("No. of pts."=w1054:i32)
              n382 = Greater?(x=w1054, y=1) -> (0:w1056:bool)
              n383 = Select(t="", s=w1056, f="For a profile the number of points should be more than 1.\n" ("Format String")) -> (s? t:f=w1052:string)
            }
            frame "Averaging:Time:(mins)" {
              n384 = Unbundle By Name(w1059) -> ("Averaging time (min)"=w1061:dbl)
              n385 = Greater Than 0?(x=w1061) -> (x > 0?=w1060:bool)
              n386 = Select(t="", s=w1060, f="The averaging time should be greater than zero.\n" ("Format String")) -> (s? t:f=w1062:string)
            }
            frame "Filename:HD:Users" {
              w1088 = FALSE  # Show Error handler
              n387 = Unbundle By Name(w1081) -> ("Filename"=w1065:path, "Row No"=w1076:i32, "Row Type Selector"=w1072:T3)
              n388 = call "Row_type_selector_string.vi"("Mode"=w1072) -> ("Output string"=w1071:string)
              n389 = call "Current_Filepath.vi"("Filename in"=w1065, "Data Type"="Results") -> ("Filename Out"=w1066:path)  [unwired: 1 out]
              n390 = Path To String(path=w1066) -> (string=w1085:string)
              n391 = Not A Number/Path/Refnum?(number/path/refnum=w1066) -> (NaN/Path/Refnum?=w1069:bool)
              n392 = Equal?(x=Multi_run_mode."Run VI Named:" ("Mode"), y=w1090) -> (x = y?=w1089:bool)
              n393 = Match Pattern(string=w1085, regular expression="-------" ("f")) -> (match substring=w1084:string)  [unwired: 4 out]
              n394 = Empty String/Path?(string/path=w1084) -> (empty?=w1070:bool)
              n395 = Format Into String(format string=" For Row  %d %s." ("Comment"), w1076, w1071) -> (resulting string=w1075:string)  [unwired: 2 in, 1 out]
              n396 = Compound Arithmetic op=AND(w1070, invert w1069) -> (w1068:bool)
              n397 = Select(t=w1066, s=w1068, f=path "") -> (s? t:f=w1083:path)
              n398 = call "Results_filename_checker.vi"("Filelength"=35, "Warn if Already Exists"=w1089, "Comment"=w1075, "Show Error handler"=w1088, "Results file"=w1083) -> ("Error String"=w1087:string, "cancelled"=w1078:bool, "Results file output"=w1080:path)  [unwired: 1 out]
              n399 = Bundle By Name(cluster=w1081, "Filename"=w1080) -> (w1079:T1)
              n400 = Not(x=w1078) -> (.not. x?=w1074:bool)
            }
            frame "No Match", Default {
              n401 = Concatenate Strings(w1094, " Has not been programmed.\n" ("string")) -> (w1092:string)
            }
          }
        }
        n402 = local read "Editted Row"() -> (w1031:bool)
        n403 = And Array Elements(Boolean array=w1027) -> (logical AND=w1026:bool)
        n404 = Concatenate Strings(w1038) -> (w1036:string)
        n405 = Concatenate Strings(w1035, w1036) -> (w1030:string)
        n406 = Empty String/Path?(string/path=w1030) -> (empty?=w1033:bool)
        n407 = case shown="True" w1033 {
          tunnel: ["Open Front Panel" w1042] -> w1032
          tunnel: w1031 -> [_ w1043]
          frame False {
          }
          frame True {
            n408 = Select(t="Close Front Panel", s=w1043, f="End") -> (s? t:f=w1042:string)
          }
        }
      }
      frame "Open Front Panel" {
        w1101 = TRUE  # Front Panel Window:Open
        n409 = Current VI's Path() -> (path=w1102:path)
        n410 = call "Open_Close_Front_Panel.ph.vi"("Front Panel Window:Open"=w1101, "VI path"=w1102) -> ()  [unwired: 2 out]
        n411 = local write "Editted Row"(TRUE ("Editted Row")) -> ()
        n412 = local write "Execution Row"(w1098) -> ()
      }
      frame "What to do next?" {
        w1112 = ""
        w1110 = "[\r\n]"
        n413 = local read "Execution Row"() -> (w1108:T1)
        n414 = Unbundle By Name(w1108) -> ("Row Type Selector"=w1124:T3, "Specific Arguments"=w1119:string, "Extra Commands"=w1117:string, "Density Ratio"=w1111:string)
        n415 = Wait Until Next ms Multiple(millisecond multiple=u32 100) -> ()  [unwired: 1 out]
        n416 = Not Equal?(x=Multi_run_mode."Blank Row" ("Mode"), y=w1124) -> (x != y?=w1120:bool)
        n417 = call "Replace_Character.vi"("Replace with"=w1112, "Input String"=w1119, "Search For"=w1110) -> ("Output string"=w1118:string)  [unwired: 1 out]
        n418 = call "Replace_Character.vi"("Replace with"=w1112, "Input String"=w1117, "Search For"=w1110) -> ("Output string"=w1116:string)  [unwired: 1 out]
        n419 = call "Replace_Character.vi"("Replace with"=w1112, "Input String"=w1111, "Search For"=w1110) -> ("Output string"=w1109:string)  [unwired: 1 out]
        n420 = Compound Arithmetic op=OR("Edit in Excel", "OK") -> (w1121:bool)
        n421 = Bundle By Name(cluster=w1108, "Specific Arguments"=w1118, "Extra Commands"=w1116, "Density Ratio"=w1109) -> (w1106:T1)
        n422 = Compound Arithmetic op=AND(w1121, w1120) -> (w1114:bool)
        n423 = Not Equal?(x=w1106, y=w1108) -> (x != y?=w1107:bool)
        n424 = Not(x="Edit in Excel") -> (.not. x?=w1105:bool)
        n425 = case shown="True" w1107 {
          tunnel: w1106 -> [_ w1128]
          frame False {
          }
          frame True {
            n426 = local write "Execution Row"(w1128) -> ()
          }
        }
        n427 = case shown="False" w1105 {
          tunnel: ["Close Front Panel" w1133] -> w1113
          tunnel: w1114 -> [_ w1132]
          frame False {
          }
          frame True {
            n428 = Select(t="Clean Up Row", s=w1132, f="What to do next?") -> (s? t:f=w1133:string)
          }
        }
        "Error Comments" <- w1115
      }
      frame "Clean Up Row" {
        n429 = call "Traverse_Control_Ch_Names.vi"("Mode"=T4."All Channel Names") -> ("Channel names"=w1142:string[])  [unwired: 1 in]
        n430 = call "Trav_Cluster_to_Row.vi"("Traverse line in"=w1137, "Row Number"=w1138, "Channel names"=w1142) -> ("Traverse line Out"=w1140:T1)  [unwired: 4 out]
      }
      frame "Close Front Panel" {
        w1146 = FALSE  # Front Panel Window:Open
        n431 = Current VI's Path() -> (path=w1147:path)
        n432 = call "Open_Close_Front_Panel.ph.vi"("Front Panel Window:Open"=w1146, "VI path"=w1147) -> ()  [unwired: 2 out]
      }
      frame "End" {
        n433 = local read "Editted Row"() -> (w1155:bool)
        n434 = case shown="True" w1155 {
          tunnel: w1154 -> [w1158 w1161]
          tunnel: [w1158 w1160] -> w1152
          tunnel: w1153 -> [_ w1159]
          frame False {
          }
          frame True {
            n435 = call "Traverse_Control_Ch_Names.vi"("Mode"=T4."All Channel Names") -> ("Channel names"=w1162:string[])  [unwired: 1 in]
            n436 = call "Trav_Cluster_to_Row.vi"("Traverse line in"=w1161, "Row Number"=w1159, "Channel names"=w1162) -> ("Traverse line Out"=w1160:T1)  [unwired: 4 out]
          }
        }
        n437 = local write "Error Comments"(w1156) -> ()
      }
    }
  }
  "Execution Row Out" <- w2
  "Continue?" <- w1
